vi "Find Resonances.vi"(8 "Error In":errorcluster, 11 "File Path Control":path=path "C:/Data/Spectra for Fedor/Ok spectra/300.00000K_175_555_2.10000V_0.00000T_May20-2015__09-37-18_001_052015.tdms") -> (0 "Error Out":errorcluster)   [LabVIEW 2016]
uses:
  <vilib>/Analysis/3filter.llb/Filter Passband Type.ctl
  <vilib>/Analysis/3filter.llb/Bessel Filter (CDB).vi
  Smooth Background CDBL.vi
  <vilib>/Analysis/NI_AALPro.lvlib
  <vilib>/Analysis/NI_AAL_SigProc.lvlib
  <vilib>/Analysis/NI_AALBase.lvlib
panel:
  out "# found":i32
  out "error":i32
  in  "Low pass distortion":dbl
  out "XY Graph 6":cluster{dbl[], dbl[]}[](graph)
  in  "User configuration":T1={"Peak width guess"=30.0, "Background removal"=enum."NONE", "Smoothing"=enum."NONE", "Smooth window"=100.0, "Relative threshold"=0.0, "Peak detector"=enum."Normal", "Bgd window"=100.0, "Spectrum recorder name"="Spectrum Recorder", "Fit window"=100.0} {"Fit window" format="%#_6pHz"; "Bgd window" format="%#_6pHz"; "Smooth window" format="%#_6pHz"; "Peak width guess" format="%#_6pHz"}
  in  "Signal channel":string="Signal"
  in  "Frequency channel":string="Frequency"
  in  "group name in":string="p"
  in  "HP F":dbl=0.1 format="%#_6p"
  in  "LP  F":dbl=0.001 format="%#_6p"
  in  "Fit?":bool
  in  "Complex":bool
  in  "Deviations":dbl=1.0
  out "variance":dbl format="%.2p"
  out "standard deviation":dbl format="%.2p"
  out "Peak F":dbl format="%#_6pHz"
  in  "Points around peak":i32=100
  in  "Peak number":i32
  out "XY Graph 5":cluster{"Array":dbl[], "Array":dbl[]}[](graph)
  out "width":i32=100 min=3
  out "XY Graph 4":cluster{"Y":dbl[], dbl[]}(graph)
  out "XY Graph 3":cluster{"Y":dbl[], "Y":dbl[]}[](graph)
  out "Magnitude":cluster{"Y":dbl[], dbl[]}[](graph)
  out "Phase":cluster{"Y":dbl[], "Unwrapped Phase":dbl[]}[](graph)
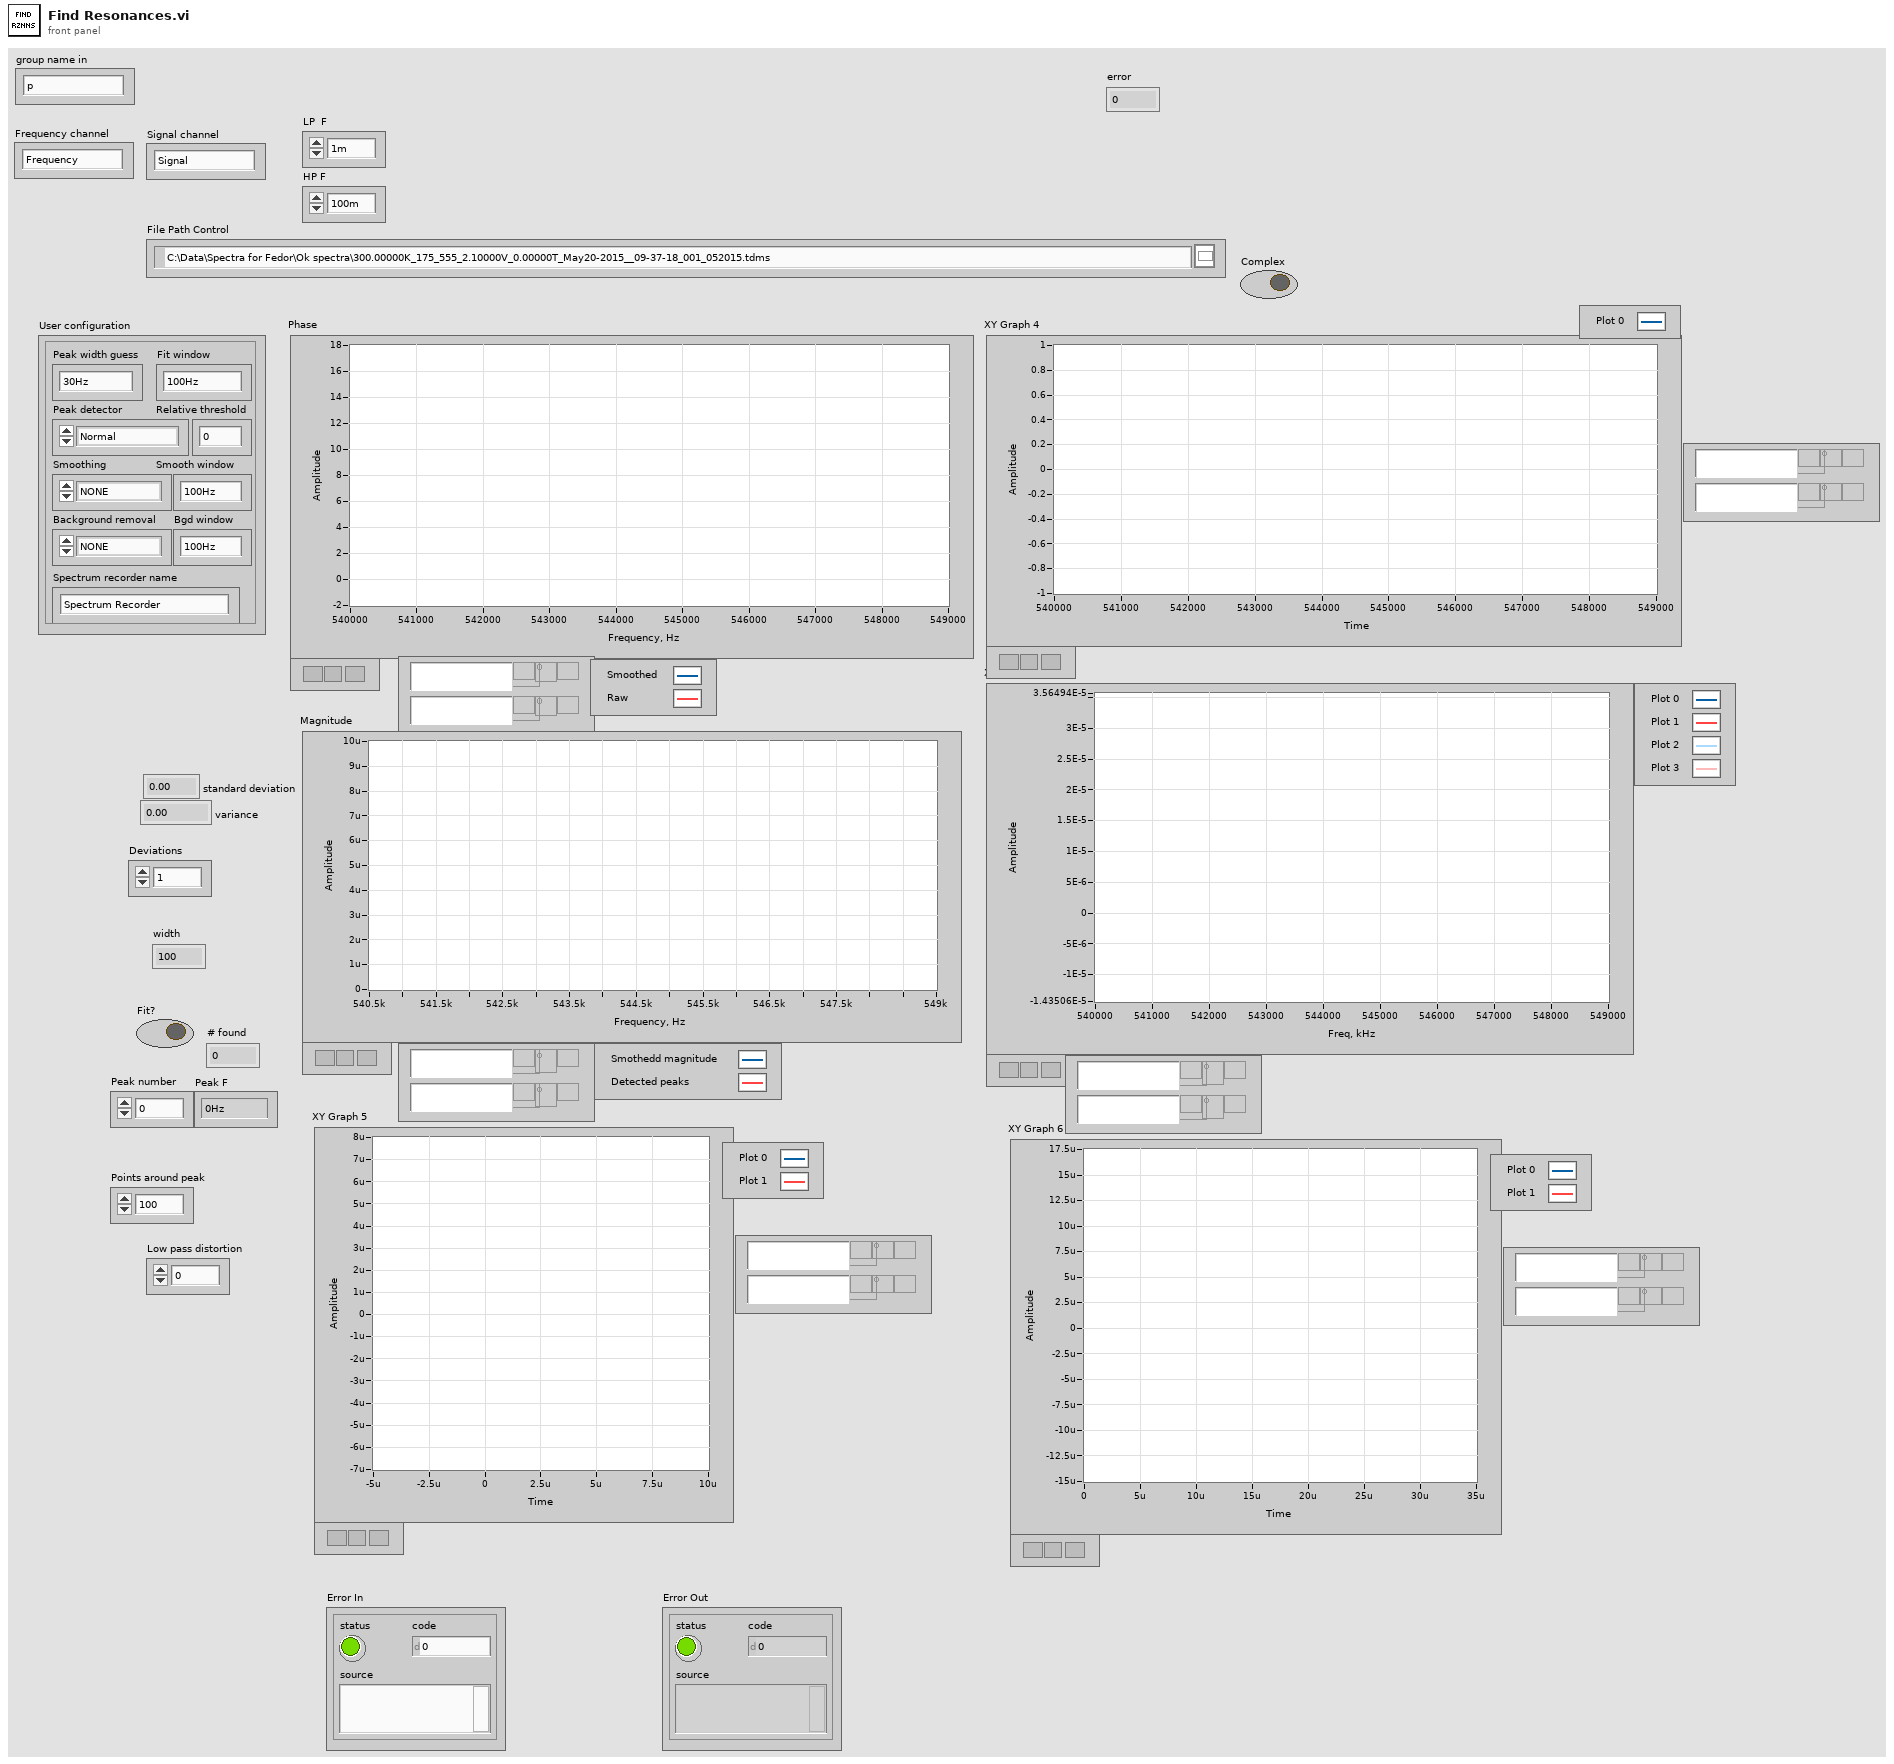
[diagram p1: front panel]
types:
  T1 = cluster{"Peak width guess":dbl, "Background removal":enum16{"NONE", "High-pass", "Detrend"}, "Smoothing":enum16{"NONE", "Low-pass", "Denoise"}, "Smooth window":dbl, "Relative threshold":dbl, "Peak detector":enum16{"Normal", "Wavelet", "Wavelet+detrend"}, "Bgd window":dbl, "Spectrum recorder name":string, "Fit window":dbl}
  T2 = enum16{"open", "open or create", "create or replace", "create", "open (read-only)"}
  T3 = typedef "NI_AALBase.lvlib/Filter Passband Type.ctl" = enum32{"Lowpass", "Highpass", "Bandpass", "Bandstop"}
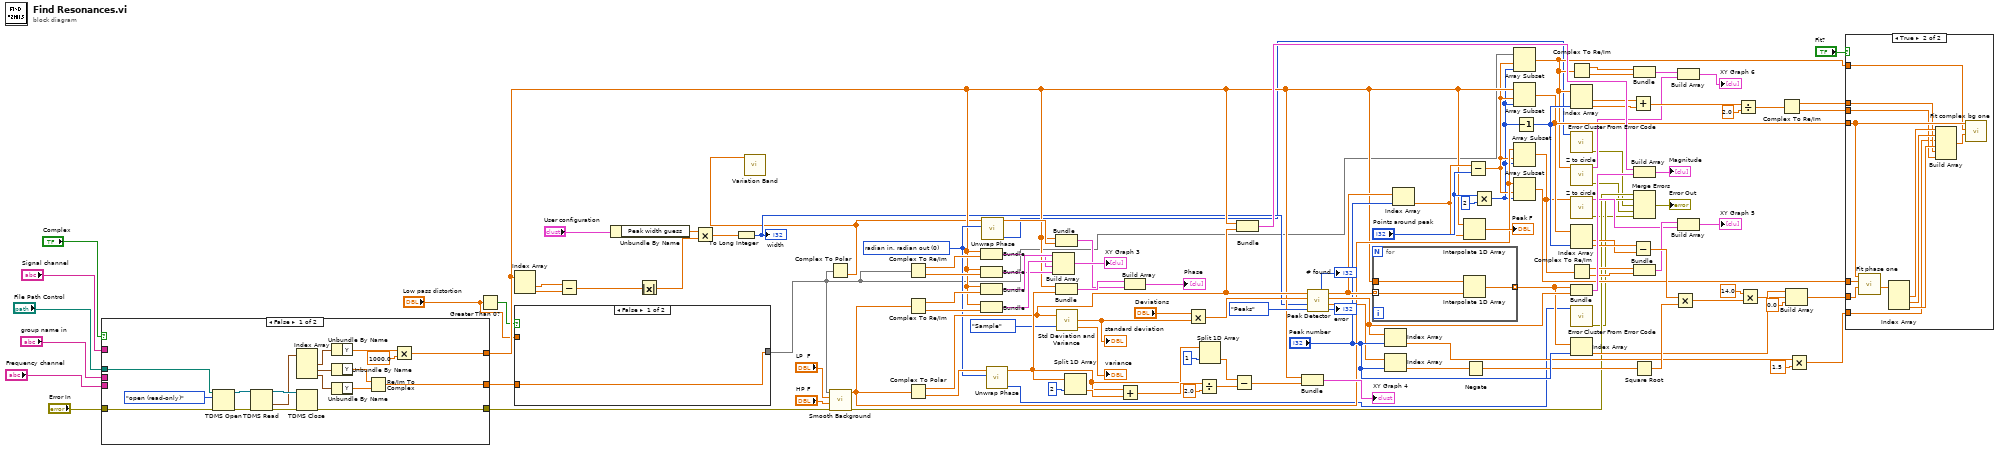
[diagram p0: block diagram]
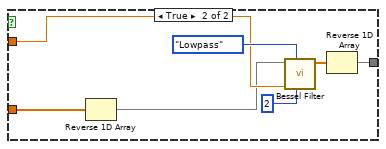
[diagram p2: hidden frame]
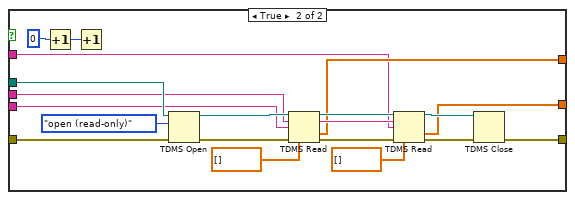
[diagram p4: hidden frame]
diagram:
  w80 = 0 items=["radian in, radian out", "radian in, degree out", "degree in, degree out", "degree in, radian out"] ("phase unit")
  n1 = case shown="False" "Complex" {
    tunnel: "File Path Control" -> [w136 w156]
    tunnel: [w120 w140] -> w39
    tunnel: "group name in" -> [_ w145]
    tunnel: "Frequency channel" -> [_ w144]
    tunnel: [w123 w141] -> w13
    tunnel: "Signal channel" -> [_ w139]
    tunnel: "Error In" -> [w122 w138]
    tunnel: [w121 w137] -> w40
    frame False {
      n2 = TDMS Open(8:w122, 10:T2."open (read-only)" ("operation (0:open)"), 11:w136) -> (0:w133:errorcluster, 3:w134:refnum<k34>)  [unwired: 4 in]
      n3 = TDMS Read(0:w134, 11:w133) -> (4:w132:refnum<k34>, 10:w130:waveform(dbl)[], 15:w131:errorcluster)  [unwired: 6 in, 3 out]
      n4 = Index Array(array=w130) -> (element #1=w129:waveform(dbl), element #2=w127:waveform(dbl), element #3=w128:waveform(dbl))  [unwired: 3 in]
      n5 = TDMS Close(8:w131, 11:w132) -> (0:w121:errorcluster)  [unwired: 1 out]
      n6 = Unbundle By Name(w129) -> ("Y"=w126:dbl[])
      n7 = Unbundle By Name(w127) -> ("Y"=w125:dbl[])
      n8 = Unbundle By Name(w128) -> ("Y"=w124:dbl[])
      n9 = Re/Im To Complex(1:w124, 2:w125) -> (0:w123:cdb[])
      n10 = Multiply(x=w126, y=1000.0) -> (x*y=w120:dbl[])
    }
    frame True {
      n11 = Increment(x=0 ("index")) -> (x+1=w150:i32)
      n12 = Increment(x=w150) -> ()  [unwired: 1 out]
      n13 = TDMS Open(8:w138, 10:T2."open (read-only)" ("operation (0:open)"), 11:w156) -> (0:w153:errorcluster, 3:w154:refnum<k34>)  [unwired: 4 in]
      n14 = TDMS Read(0:w154, 5:w145, 7:w144, 11:w153, 12:dbl[] []) -> (4:w148:refnum<k34>, 6:w146:string, 10:w140:dbl[], 15:w152:errorcluster)  [unwired: 3 in, 2 out]
      n15 = TDMS Read(0:w148, 5:w146, 7:w139, 11:w152, 12:cdb[] []) -> (4:w147:refnum<k34>, 10:w141:cdb[], 15:w149:errorcluster)  [unwired: 3 in, 3 out]
      n16 = TDMS Close(8:w149, 11:w147) -> (0:w137:errorcluster)  [unwired: 1 out]
    }
  }
  n17 = Greater Than 0?(x="Low pass distortion") -> (x > 0?=w15:bool)
  n18 = Index Array(array=w39) -> (element #1=w38:dbl, element #2=w37:dbl)  [unwired: 2 in]
  n19 = case shown="False" w15 {
    tunnel: w13 -> [w157 w164]
    tunnel: [w157 w158] -> w12
    tunnel: "Low pass distortion" -> [_ w161]
    frame False {
    }
    frame True {
      n20 = Reverse 1D Array(array=w164) -> (reversed array=w159:cdb[])
      n21 = call-poly <vilib>:"Bessel Filter.vi"("order"=2, "filter type"=Filter_Passband_Type."Lowpass", "low cutoff freq: fl"=w161, "X"=w159) -> ("Filtered X"=w163:cdb[])  [unwired: 4 in, 1 out]
      n22 = Reverse 1D Array(array=w163) -> (reversed array=w158:cdb[])
    }
  }
  n23 = Subtract(x=w38, y=w37) -> (x-y=w36:dbl)
  n24 = Unbundle By Name("User configuration") -> ("Peak width guess"=w34:dbl)
  n25 = Absolute Value(x=w36) -> (abs(x)=w33:dbl)
  n26 = Multiply(x=w34, y=w33) -> (x*y=w32:dbl)
  n27 = To Long Integer(number=w32) -> (32bit integer=w31:i32)
  "width" <- w31
  n28 = Complex To Polar(r * e^(i*theta)=w12) -> (theta=w1:dbl[])  [unwired: 1 out]
  n29 = call "Variation Band.vi"("Data"=w1) -> ()  [unwired: 11 in]
  n30 = call-poly "Smooth Background.vi"("Error In"=w40, "HP F"="HP F", "LP  F"="LP  F", "Data"=w12) -> ("Error Out"=w11:errorcluster, "Data out"=w51:cdb[])  [unwired: 6 in]
  n31 = Complex To Re/Im(x + iy=w12) -> (x=w90:dbl[], y=w91:dbl[])
  n32 = Complex To Re/Im(x + iy=w51) -> (x=w102:dbl[], y=w101:dbl[])
  n33 = Complex To Polar(r * e^(i*theta)=w51) -> (r=w87:dbl[], theta=w108:dbl[])
  n34 = Bundle(w39, w90) -> (w89:cluster{dbl[], dbl[]})  [unwired: 1 in]
  n35 = Bundle(w39, w91) -> (w88:cluster{dbl[], dbl[]})  [unwired: 1 in]
  n36 = Bundle(w39, w102) -> (w116:cluster{dbl[], dbl[]})  [unwired: 1 in]
  n37 = Bundle(w39, w101) -> (w115:cluster{dbl[], dbl[]})  [unwired: 1 in]
  n38 = call <vilib>:"Unwrap Phase.vi"("phase unit"=w80, "Phase"=w1) -> ("error"=w9:i32, "Unwrapped Phase"=w79:dbl[])  [unwired: 8 in]
  n39 = call <vilib>:"Unwrap Phase.vi"("phase unit"=w80, "Phase"=w108) -> ("error"=w10:i32, "Unwrapped Phase"=w103:dbl[])  [unwired: 8 in]
  n40 = Build Array(w116, w115, w89, w88) -> (→"XY Graph 3":cluster{dbl[], dbl[]}[])
  n41 = Bundle(w39, "Unwrapped Phase"=w79) -> (w77:cluster{dbl[], "Unwrapped Phase":dbl[]})  [unwired: 1 in]
  n42 = Bundle(w39, "Unwrapped Phase"=w103) -> (w117:cluster{dbl[], "Unwrapped Phase":dbl[]})  [unwired: 1 in]
  n43 = call <vilib>:"Std Deviation and Variance.vi"("X"=w87, "Weighting (Sample)"=enum16{"Sample", "Population"}."Sample") -> ("standard deviation"=w82:dbl, "variance"=→"variance":dbl)  [unwired: 1 out]
  "standard deviation" <- w82
  n44 = Split 1D Array(array=w103, index=2) -> (second subarray=w111:dbl[])  [unwired: 1 out]
  n45 = Add(x=w103, y=w111) -> (x+y=w110:dbl[])
  n46 = Build Array(w117, w77) -> (→"Phase":cluster{dbl[], "Unwrapped Phase":dbl[]}[])
  n47 = Multiply(x="Deviations", y=w82) -> (x*y=w83:dbl)
  n48 = Divide(x=w110, y=2.0) -> (x/y=w107:dbl[])
  n49 = Split 1D Array(array=w103, index=1) -> (second subarray=w104:dbl[])  [unwired: 1 out]
  n50 = Subtract(x=w104, y=w107) -> (x-y=w106:dbl[])
  n51 = Bundle(w39, w87) -> (w100:cluster{dbl[], dbl[]})  [unwired: 1 in]
  n52 = Bundle(w39, w106) -> (→"XY Graph 4":cluster{dbl[], dbl[]})  [unwired: 1 in]
  n53 = call <vilib>:"Peak Detector.vi"("peaks/valleys"=enum32{"Peaks", "Valleys"}."Peaks", "width"=w31, "threshold"=w83, "X"=w87) -> ("error"=→"error":i32, "2nd Derivatives"=w67:dbl[], "Amplitudes"=w74:dbl[], "Locations"=w69:dbl[], "# found"=→"# found":i32)  [unwired: 3 in]
  n54 = for {
    tunnel: w39 -> [w167]
    tunnel: w69 -> [w166] mode=indexing
    tunnel: [w165] -> w73 mode=indexing
    n55 = Interpolate 1D Array(1:w166, 2:w167) -> (0:w165:dbl)
  }
  n56 = Index Array(array=w74, index="Peak number") -> (element=w46:dbl)
  n57 = Index Array(array=w67, index="Peak number") -> (element=w66:dbl)
  n58 = Index Array(array=w69, index="Peak number") -> (element=w75:dbl)
  n59 = Interpolate 1D Array(1:w75, 2:w39) -> (0:→"Peak F":dbl)
  n60 = Negate(x=w66) -> (-x=w63:dbl)
  n61 = Subtract(x=w75, y="Points around peak") -> (x-y=w28:dbl)
  n62 = Multiply(x="Points around peak", y=2) -> (x*y=w27:i32)
  n63 = Array Subset(array=w12, index=w28, length=w27) -> (w21:cdb[])
  n64 = Array Subset(array=w39, index=w28, length=w27) -> (w26:dbl[])
  n65 = Array Subset(array=w51, index=w28, length=w27) -> (w19:cdb[])
  n66 = Array Subset(array=w51, index=w28, length=w27) -> (w52:cdb[])
  n67 = Decrement(x=w27) -> (x-1=w72:i32)
  n68 = Index Array(array=w21, index #2=w72) -> (element #1=w62:cdb, element #2=w61:cdb)  [unwired: 1 in]
  n69 = call <vilib>:"Error Cluster From Error Code.vi"("error code (0)"=w9) -> ("error out"=w6:errorcluster)  [unwired: 8 in]
  n70 = call "Z to circle.vi"("Z"=w21) -> ("Error Out"=w5:errorcluster, "plot"=w20:cluster{"Array":dbl[], "Array":dbl[]})  [unwired: 4 in, 5 out]
  n71 = call "Z to circle.vi"("Z"=w19) -> ("Error Out"=w4:errorcluster, "plot"=w17:cluster{"Array":dbl[], "Array":dbl[]})  [unwired: 4 in, 5 out]
  n72 = Index Array(array=w26, index #2=w72) -> (element #1=w70:dbl, element #2=w71:dbl)  [unwired: 1 in]
  n73 = Bundle(w73, "Amplitudes"=w74) -> (w97:cluster{dbl[], "Amplitudes":dbl[]})  [unwired: 1 in]
  n74 = call <vilib>:"Error Cluster From Error Code.vi"("error code (0)"=w10) -> ("error out"=w7:errorcluster)  [unwired: 8 in]
  n75 = Index Array(array=w73, index="Peak number") -> (element=w59:dbl)
  n76 = Complex To Re/Im(x + iy=w21) -> (x=w24:dbl[], y=w23:dbl[])
  n77 = Complex To Re/Im(x + iy=w19) -> (x=w94:dbl[], y=w93:dbl[])
  n78 = Add(x=w62, y=w61) -> (x+y=w60:cdb)
  n79 = Subtract(x=w71, y=w70) -> (x-y=w64:dbl)
  n80 = Square Root(x=w63) -> (sqrt(x)=w65:dbl)
  n81 = Bundle(w24, w23) -> (w25:cluster{dbl[], dbl[]})  [unwired: 1 in]
  n82 = Build Array(w100, w97) -> (→"Magnitude":cluster{dbl[], "Amplitudes":dbl[]}[])
  n83 = Merge Errors(w11, w7, w6, w5, w4) -> (→"Error Out":errorcluster)
  n84 = Bundle(w94, w93) -> (w18:cluster{dbl[], dbl[]})  [unwired: 1 in]
  n85 = Multiply(x=w64, y=w65) -> (x*y=w58:dbl)
  n86 = Build Array(w25, w20) -> (→"XY Graph 6":cluster{"Array":dbl[], "Array":dbl[]}[])
  n87 = Build Array(w18, w17) -> (→"XY Graph 5":cluster{"Array":dbl[], "Array":dbl[]}[])
  n88 = Divide(x=w60, y=2.0) -> (x/y=w55:cdb)
  n89 = Multiply(x=14.0, y=w58) -> (x*y=w30:dbl)
  n90 = Complex To Re/Im(x + iy=w55) -> (x=w54:dbl, y=w53:dbl)
  n91 = Build Array(w59, w30, 0.0 ("element")) -> (w56:dbl[])
  n92 = Multiply(x=w46, y=1.5) -> (x*y=w45:dbl)
  n93 = case shown="True" "Fit?" {
    tunnel: w21 -> [_ w178]
    tunnel: w26 -> [_ w179]
    tunnel: w56 -> [_ w177]
    tunnel: w45 -> [_ w169]
    tunnel: w54 -> [_ w172]
    tunnel: w53 -> [_ w171]
    tunnel: w52 -> [_ w168]
    frame False {
    }
    frame True {
      n94 = call "Fit phase one.vi"("Initial parameters"=w177, "Z"=w168, "X"=w179) -> ("best fit parameters"=w176:dbl[])  [unwired: 7 in, 1 out]
      n95 = Index Array(array=w176) -> (element #1=w175:dbl, element #2=w174:dbl, element #3=w173:dbl)  [unwired: 3 in]
      n96 = Build Array(w175, w174, w169, w173, w172, w171) -> (w170:dbl[])
      n97 = call "Fit complex bg one.vi"("Initial parameters"=w170, "Z"=w178, "X"=w179) -> ()  [unwired: 6 in, 3 out]
    }
  }
